vi "DIAdem Daemon.vi"(8 "error in (no error)":errorcluster, 10 "Queues":T2, 11 "DIAdem Reference":T1) -> (0 "error out":errorcluster, 2 "dup Queues":T2, 3 "dup DIAdem Reference":T1)   [LabVIEW 2011]
uses:
  lib/DIAdem Queues.ctl
  lib/DIAdem Daemon Queue.ctl
  lib/DIAdem Daemon Script Type.ctl
  Datasheet/Datasheet Inputs.ctl
  www/cgi-bin/_cgi-lib/TDM_INDEX Record.ctl
  Datasheet/Datasheet Generator Settings.ctl
  www/cgi-bin/runtest/runtest Queue.ctl
  www/tests/Test Output.ctl
  database/Fields/Field Record.ctl
  database/Fields/Field DataTypes.ctl
  database/Fields/Field NextItem.ctl
  <vilib>/ExportToExcel/DIAdem Reference.ctl
panel:
  in  "local DIAdem Reference":T1
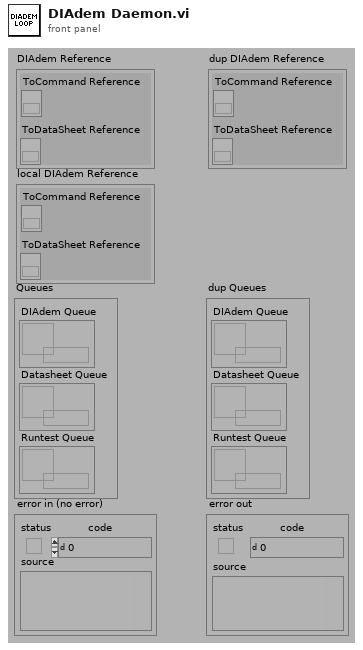
[diagram p1: front panel]
types:
  T1 = typedef "DIAdem Reference.ctl" = cluster{"ToCommand Reference":refnum<k7>, "ToDataSheet Reference":refnum<k7>}
  T2 = typedef "DIAdem Queues.ctl" = cluster{"DIAdem Queue":refnum<queue>, "Datasheet Queue":refnum<queue>, "Runtest Queue":refnum<queue>}
  T3 = typedef "DIAdem Daemon Queue.ctl" = cluster{"Report Template TDM":path, "Report Processor VBS":path, "Report Path PDF":path, "Report Script Params":string, "Username":string, "Script Type":T4, "Report Query Params":string, "Client Machine":string, "Print on Client?":bool, "Response Queue Name":string, "Script Variables":string[], "Start Request Time":timestamp, "Wait?":bool}
  T4 = typedef "DIAdem Daemon Script Type.ctl" = enum16{"Report", "Query", "Script", "Datasheet", "Append", "Restart", "Stop"}
  T5 = cluster{"ToCommand Reference":bool, "ToDataSheet Reference":bool}
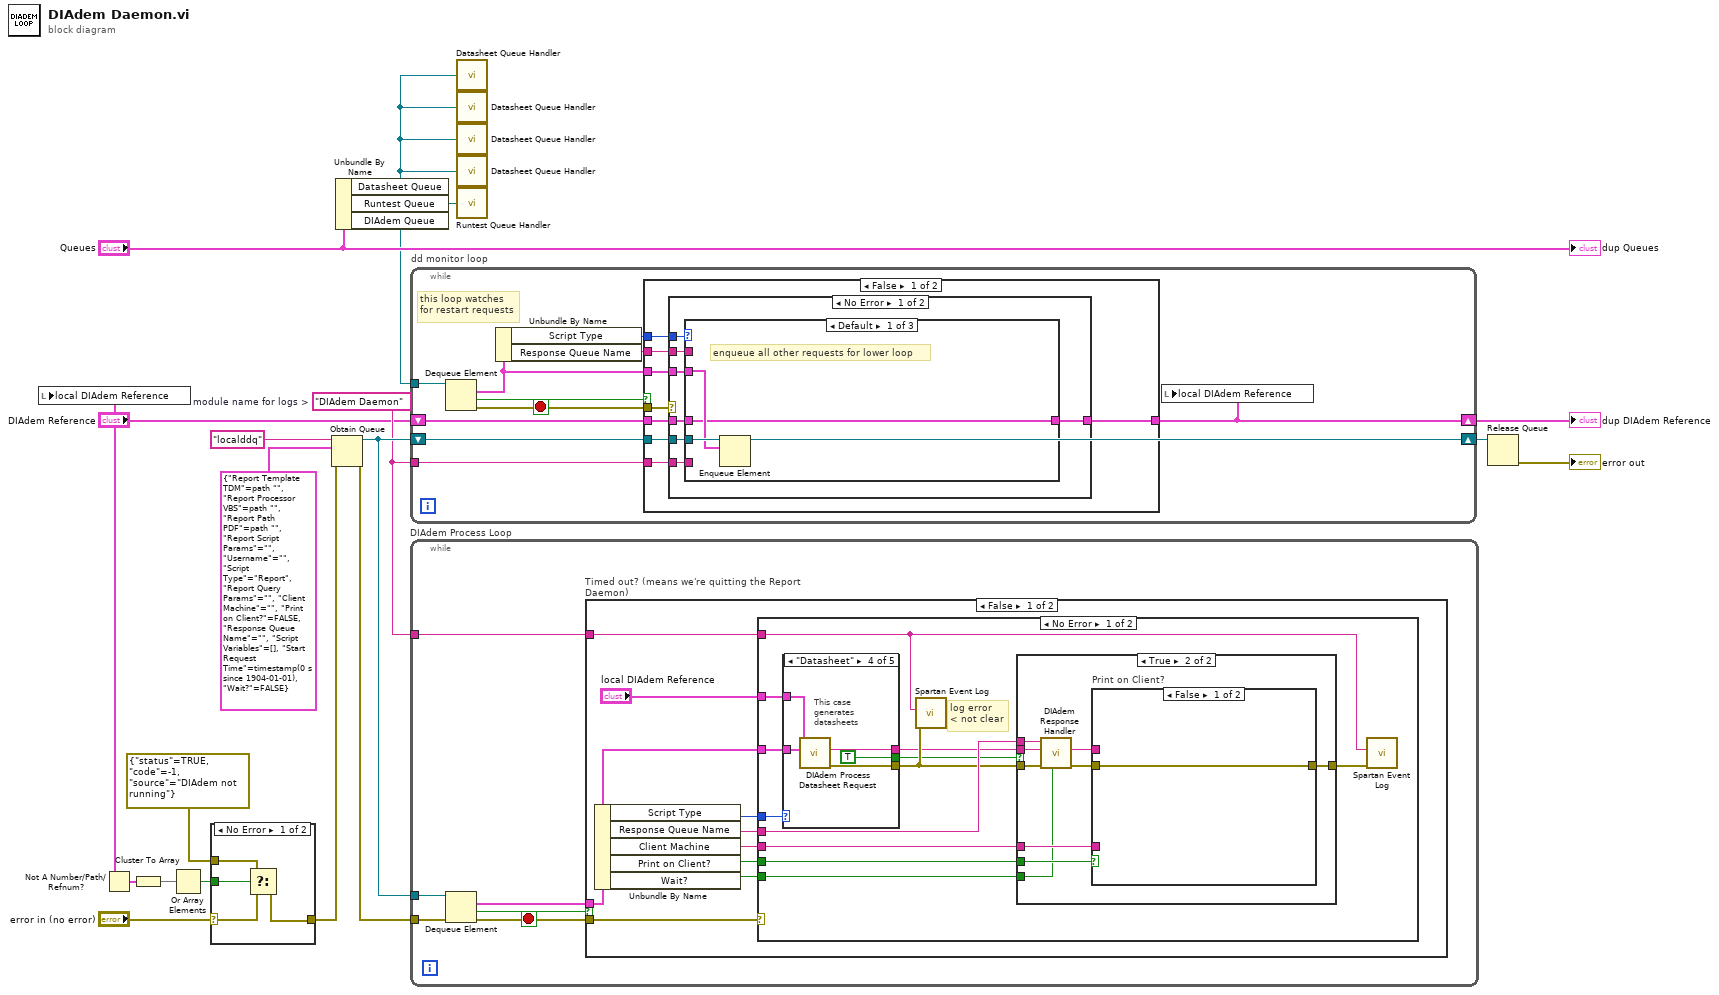
[diagram p0: block diagram]
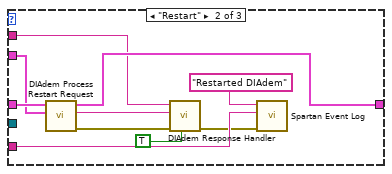
[diagram p2: hidden frame]
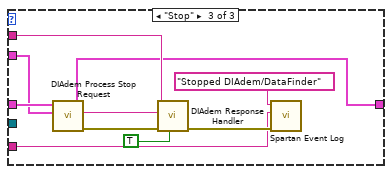
[diagram p3: hidden frame]
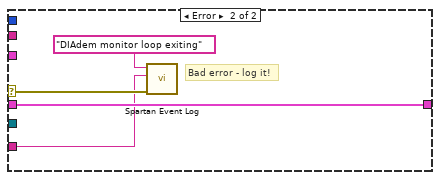
[diagram p4: hidden frame]
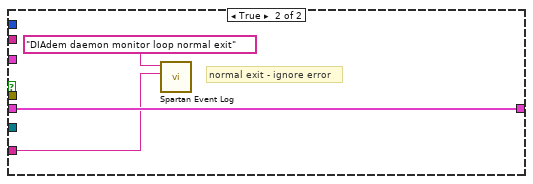
[diagram p5: hidden frame]
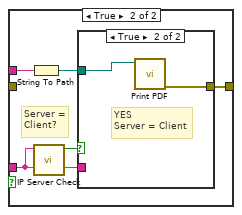
[diagram p8: hidden frame]
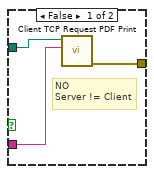
[diagram p9: hidden frame]
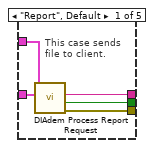
[diagram p10: hidden frame]
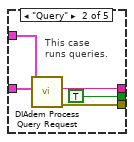
[diagram p11: hidden frame]
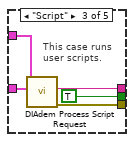
[diagram p12: hidden frame]
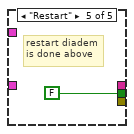
[diagram p13: hidden frame]
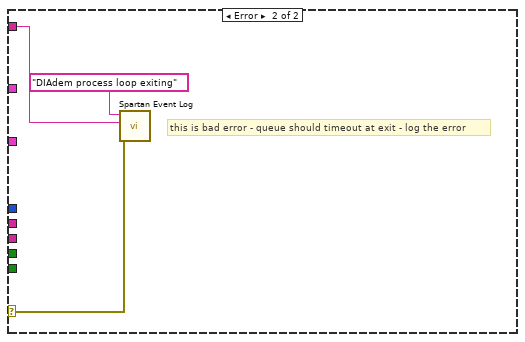
[diagram p14: hidden frame]
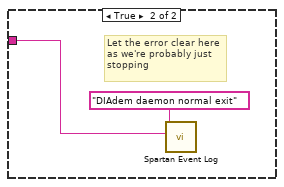
[diagram p15: hidden frame]
diagram:
  w8 = "DIAdem Daemon"  # module name for logs >
  n1 = local write "local DIAdem Reference"("DIAdem Reference") -> ()
  n2 = Not A Number/Path/Refnum?(number/path/refnum="DIAdem Reference") -> (NaN/Path/Refnum?=w19:T5)
  n3 = Cluster To Array(cluster=w19) -> (array=w18:bool[])
  n4 = Or Array Elements(Boolean array=w18) -> (logical OR=w17:bool)
  n5 = case shown="No Error" "error in (no error)" {
    selector: "error in (no error)" -> [w22 w24]
    tunnel: w17 -> [w23 _]
    tunnel: [w21 w24] -> w13
    tunnel: errorcluster {"status"=TRUE, "code"=-1, "source"="DIAdem not running"} ("error IN") -> [w20 _]
    frame No Error {
      n6 = Select(t=w20, s=w23, f=w22) -> (s? t:f=w21:errorcluster)
    }
    frame Error {
    }
  }
  n7 = Obtain Queue(name (unnamed)="localddq", element data type=T3 {"Report Template TDM"=path "", "Report Processor VBS"=path "", "Report Path PDF"=path "", "Report Script Params"="", "Username"="", "Script Type"=enum."Report", "Report Query Params"="", "Client Machine"="", "Print on Client?"=FALSE, "Response Queue Name"="", "Script Variables"=[], "Start Request Time"=timestamp(0 s since 1904-01-01), "Wait?"=FALSE} ("DIAdem Queue"), error in (no error)=w13) -> (queue out=w11:refnum<queue>, error out=w12:errorcluster)  [unwired: 2 in, 1 out]
  n8 = Unbundle By Name("Queues") -> ("Datasheet Queue"=w2:refnum<queue>, "Runtest Queue"=w3:refnum<queue>, "DIAdem Queue"=w1:refnum<queue>)
  n9 = while "dd monitor loop" {
    tunnel: w1 -> [w34]
    shift-right: [w29] -> w9
    shift-left: "DIAdem Reference" -> [w32]
    shift-right: [w28] -> w10
    shift-left: w11 -> [w28]
    tunnel: w8 -> [w25]
    stop <- w26 stop-if-true
    # "this loop watches\nfor restart requests"
    n10 = Dequeue Element(queue=w34) -> (element=w31:T3, timed out?=w27:bool, error out=w26:errorcluster)  [unwired: 1 in, 2 out]
    n11 = Unbundle By Name(w31) -> ("Script Type"=w33:T4, "Response Queue Name"=w30:string)
    n12 = case shown="False" w27 {
      tunnel: w33 -> [w42 _]
      tunnel: w32 -> [w41 w79]
      tunnel: w31 -> [w40 _]
      tunnel: w28 -> [w39 _]
      tunnel: w30 -> [w38 _]
      tunnel: [w37 w79] -> w29
      tunnel: w26 -> [w36 _]
      tunnel: w25 -> [w35 w77]
      frame False {
        n13 = case shown="No Error" w36 {
          selector: w36 -> [_ w75]
          tunnel: w42 -> [w49 _]
          tunnel: w41 -> [w48 w74]
          tunnel: w40 -> [w47 _]
          tunnel: w39 -> [w46 _]
          tunnel: w38 -> [w45 _]
          tunnel: [w44 w74] -> w37
          tunnel: w35 -> [w43 w73]
          frame No Error {
            n14 = case shown="Default" w49 {
              tunnel: w48 -> [w50 w62 w72]
              tunnel: w47 -> [w51 w61 w71]
              tunnel: w46 -> [w52 _ _]
              tunnel: w45 -> [_ w56 w67]
              tunnel: [w50 w60 w65] -> w44
              tunnel: w43 -> [_ w58 w64]
              frame Default {
                # "enqueue all other requests for lower loop"
                n15 = Enqueue Element(queue=w52, element=w51) -> ()  [unwired: 1 in, 4 out]
              }
              frame "Restart" {
                n16 = call "DIAdem Process Restart Request.vi"("DIAdem Queue"=w61, "DIAdem Reference"=w62) -> ("error out"=w54:errorcluster, "Script Result"=w55:string, "DIAdem Reference"=w60:T1)  [unwired: 1 in, 3 out]
                n17 = call "DIAdem Response Handler.vi"("Wait? (T)"=TRUE, "error in (no error)"=w54, "Response String (\"\")"=w55, "Response Queue Name (\"\")"=w56) -> ("error out"=w57:errorcluster)  [unwired: 7 out]
                n18 = call "Spartan Event Log.vi"("error in (no error)"=w57, "module (\"\")"=w58, "message (\"\")"="Restarted DIAdem" ("message (\"\")")) -> ()  [unwired: 2 in, 4 out]
              }
              frame "Stop" {
                n19 = call "DIAdem Process Stop Request.vi"("DIAdem Queue"=w71, "DIAdem Reference"=w72) -> ("error out"=w66:errorcluster, "Script Result"=w68:string, "DIAdem Reference"=w65:T1)  [unwired: 1 in, 3 out]
                n20 = call "DIAdem Response Handler.vi"("Wait? (T)"=TRUE ("Wait?"), "error in (no error)"=w66, "Response String (\"\")"=w68, "Response Queue Name (\"\")"=w67) -> ("error out"=w70:errorcluster)  [unwired: 7 out]
                n21 = call "Spartan Event Log.vi"("error in (no error)"=w70, "module (\"\")"=w64, "message (\"\")"="Stopped DIAdem/DataFinder" ("message (\"\")")) -> ()  [unwired: 2 in, 4 out]
              }
            }
          }
          frame Error {
            # "Bad error - log it!"
            n22 = call "Spartan Event Log.vi"("error in (no error)"=w75, "module (\"\")"=w73, "message (\"\")"="DIAdem monitor loop exiting" ("name (unnamed)")) -> ()  [unwired: 2 in, 4 out]
          }
        }
      }
      frame True {
        # "normal exit - ignore error"
        n23 = call "Spartan Event Log.vi"("module (\"\")"=w77, "message (\"\")"="DIAdem daemon monitor loop normal exit" ("message (\"\")")) -> ()  [unwired: 3 in, 4 out]
      }
    }
    n24 = local write "local DIAdem Reference"(w29) -> ()
  }
  "dup DIAdem Reference" <- w9
  n25 = while "DIAdem Process Loop" {
    tunnel: w12 -> [w85]
    tunnel: w11 -> [w81]
    tunnel: w8 -> [w80]
    stop <- w83 stop-if-true
    n26 = Dequeue Element(queue=w81, error in (no error)=w85) -> (element=w84:T3, timed out?=w82:bool, error out=w83:errorcluster)  [unwired: 2 out]
    n27 = case "Timed out? (means we're quitting the Report Daemon)" shown="False" w82 {
      tunnel: w84 -> [w94 _]
      tunnel: w83 -> [w91 _]
      tunnel: w80 -> [w87 w153]
      frame False {
        n28 = Unbundle By Name(w94) -> ("Script Type"=w93:T4, "Response Queue Name"=w92:string, "Client Machine"=w90:string, "Print on Client?"=w89:bool, "Wait?"=w86:bool)
        n29 = case shown="No Error" w91 {
          selector: w91 -> [_ w150]
          tunnel: "local DIAdem Reference" -> [w106 _]
          tunnel: w94 -> [w105 _]
          tunnel: w93 -> [w104 _]
          tunnel: w92 -> [w103 _]
          tunnel: w90 -> [w98 _]
          tunnel: w89 -> [w99 _]
          tunnel: w87 -> [w96 w149]
          tunnel: w86 -> [w95 _]
          frame No Error {
            # "log error\n< not clear"
            n30 = case shown="\"Datasheet\"" w104 {
              tunnel: w106 -> [w132 w137 w142 w147 _]
              tunnel: w105 -> [w131 w136 w141 w146 _]
              tunnel: [w130 w135 w140 w145 _] -> w102
              tunnel: [w129 w134 w139 w144 _] -> w101
              tunnel: [w128 TRUE ("Done?") TRUE ("Done?") TRUE ("Done?") FALSE ("Done?")] -> w100
              frame "Report", Default {
                # "This case sends\nfile to client."
                n31 = call "DIAdem Process Report Request.vi"("DIAdem Queue"=w131, "DIAdem Reference"=w132) -> ("error out"=w130:errorcluster, "Done?"=w128:bool, "Output"=w129:string)  [unwired: 2 in, 5 out]
              }
              frame "Query" {
                # "This case\nruns queries."
                n32 = call "DIAdem Process Query Request.vi"("DIAdem Queue"=w136, "DIAdem Reference"=w137) -> ("error out"=w135:errorcluster, "Results"=w134:string)  [unwired: 1 in, 4 out]
              }
              frame "Script" {
                # "This case runs \nuser scripts."
                n33 = call "DIAdem Process Script Request.vi"("DIAdem Queue"=w141, "DIAdem Reference"=w142) -> ("error out"=w140:errorcluster, "Script Result"=w139:string)  [unwired: 1 in, 4 out]
              }
              frame "Datasheet" {
                # "This case\ngenerates\ndatasheets"
                n34 = call "DIAdem Process Datasheet Request.vi"("DIAdem Queue"=w146, "DIAdem Reference"=w147) -> ("error out"=w145:errorcluster, "Script Result"=w144:string)  [unwired: 1 in, 4 out]
              }
              frame "Restart" {
                # "restart diadem\nis done above"
              }
            }
            n35 = call "Spartan Event Log.vi"("error in (no error)"=w102, "module (\"\")"=w96) -> ()  [unwired: 3 in, 4 out]
            n36 = case shown="True" w100 {
              tunnel: w103 -> [_ w113]
              tunnel: [w107 w116] -> w97
              tunnel: w102 -> [w107 w109]
              tunnel: w101 -> [_ w112]
              tunnel: w99 -> [_ w115]
              tunnel: w98 -> [_ w114]
              tunnel: w95 -> [_ w108]
              frame False {
              }
              frame True {
                n37 = call "DIAdem Response Handler.vi"("Wait? (T)"=w108, "error in (no error)"=w109, "Response String (\"\")"=w112, "Response Queue Name (\"\")"=w113) -> ("error out"=w110:errorcluster, "Response String"=w111:string)  [unwired: 6 out]
                n38 = case "Print on Client?" shown="False" w115 {
                  tunnel: w110 -> [w117 _]
                  tunnel: [w117 w122] -> w116
                  tunnel: w111 -> [_ w118]
                  tunnel: w114 -> [_ w119]
                  frame False {
                  }
                  frame True {
                    # "Server =\nClient?"
                    n39 = String To Path(string=w118) -> (path=w121:path)
                    n40 = call "IP Server Check.vi"("IP Address"=w119) -> ("IP Same as execution Computer?"=w120:bool)  [unwired: 10 out]
                    n41 = case shown="True" w120 {
                      tunnel: [w124 w126] -> w122
                      tunnel: w119 -> [w123 _]
                      tunnel: w121 -> [w125 w127]
                      frame False {
                        # "NO\nServer != Client"
                        n42 = call "Client TCP Request PDF Print.vi"("Client (\"\": localhost)"=w123, "Report PDF Path"=w125) -> ("error out"=w124:errorcluster)  [unwired: 1 in, 8 out]
                      }
                      frame True {
                        # "YES\nServer = Client"
                        n43 = call "Print PDF.vi"("PDF Path"=w127) -> ("error out"=w126:errorcluster)  [unwired: 1 in, 9 out]
                      }
                    }
                  }
                }
              }
            }
            n44 = call "Spartan Event Log.vi"("error in (no error)"=w97, "module (\"\")"=w96) -> ()  [unwired: 3 in, 4 out]
          }
          frame Error {
            # "this is bad error - queue should timeout at exit - log the error"
            n45 = call "Spartan Event Log.vi"("error in (no error)"=w150, "module (\"\")"=w149, "message (\"\")"="DIAdem process loop exiting" ("name (unnamed)")) -> ()  [unwired: 2 in, 4 out]
          }
        }
      }
      frame True {
        # "Let the error clear here\nas we're probably just\nstopping"
        n46 = call "Spartan Event Log.vi"("module (\"\")"=w153, "message (\"\")"="DIAdem daemon normal exit" ("name (unnamed)")) -> ()  [unwired: 3 in, 4 out]
      }
    }
  }
  n47 = call "Datasheet Queue Handler.vi"("Datasheet Queue"=w2) -> ()
  n48 = call "Datasheet Queue Handler.vi"("Datasheet Queue"=w2) -> ()
  n49 = call "Datasheet Queue Handler.vi"("Datasheet Queue"=w2) -> ()
  n50 = call "Datasheet Queue Handler.vi"("Datasheet Queue"=w2) -> ()
  n51 = call "Runtest Queue Handler.vi"("Runtest Queue"=w3) -> ()
  n52 = Release Queue(queue=w10) -> (error out=→"error out":errorcluster)  [unwired: 1 in, 3 out]
  "dup Queues" <- "Queues"
